vi "Quit.vi"(0 "reference in":refnum<class "RedisConnection.lvclass">, 11 "Error In":errorcluster) -> (4 "reference out":refnum<class "RedisConnection.lvclass">, 8 "Data":T1, 15 "Error Out":errorcluster)   [LabVIEW 2020, in "RedisConnection.lvclass"]
uses:
  RedisConnection.lvclass
  RedisDataType.ctl
  ReplyDataTypeEnum.ctl
  RedisConnection.lvclass/RedisConnection.ctl
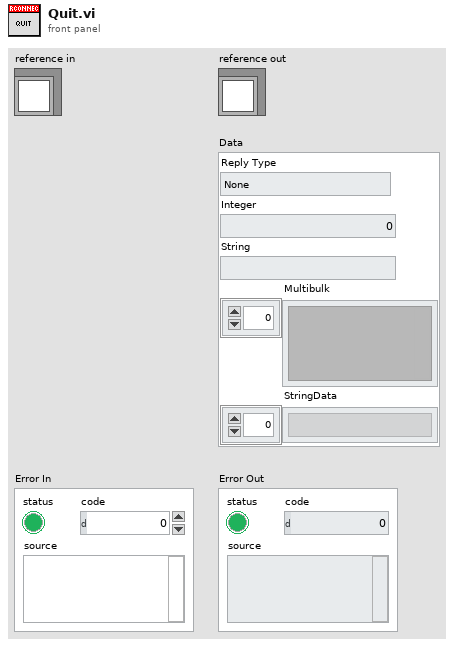
[diagram p1: front panel]
types:
  T1 = typedef "RedisConnection.lvclass/RedisDataType.ctl" = cluster{"Reply Type":T2, "Integer":i64, "String":string, "Multibulk":variant[], "StringData":string[]}
  T2 = typedef "RedisConnection.lvclass/ReplyDataTypeEnum.ctl" = enum16{"None", "Error", "Status", "Nil", "Integer", "String", "Multibulk"}
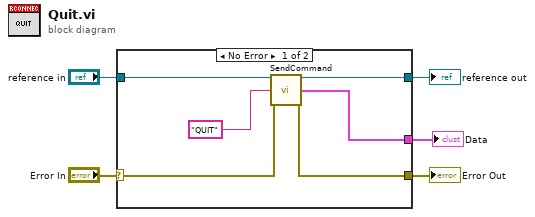
[diagram p0: block diagram]
diagram:
  n1 = case shown="No Error" "Error In" {
    selector: "Error In" -> [w9 w13]
    tunnel: [w8 w13] -> w4
    tunnel: [w11 w12] -> w2
    tunnel: "reference in" -> [w10 w12]
    tunnel: [w6 _] -> w1
    frame No Error {
      n2 = call "SendCommand.vi"("reference in"=w10, "Command"="QUIT", "Error In"=w9) -> ("reference out"=w11:refnum<class "RedisConnection.lvclass">, "Data"=w6:T1, "Error Out"=w8:errorcluster)  [unwired: 10 in]
    }
    frame Error {
    }
  }
  "Error Out" <- w4
  "reference out" <- w2
  "Data" <- w1
